vi "Controlar brazo.vi"() -> (3 "fin":bool)   [LabVIEW 2018]
panel:
  in  "Stop Button":bool
  out "Elapsed Time (s) 2":dbl
  out "Tiempo \ntranscurrido (s) 2":dbl caption="Elapsed Time (s)"
  out "Elapsed Time (s)":dbl
  out "Tiempo \ntranscurrido (s)":dbl caption="Elapsed Time (s)"
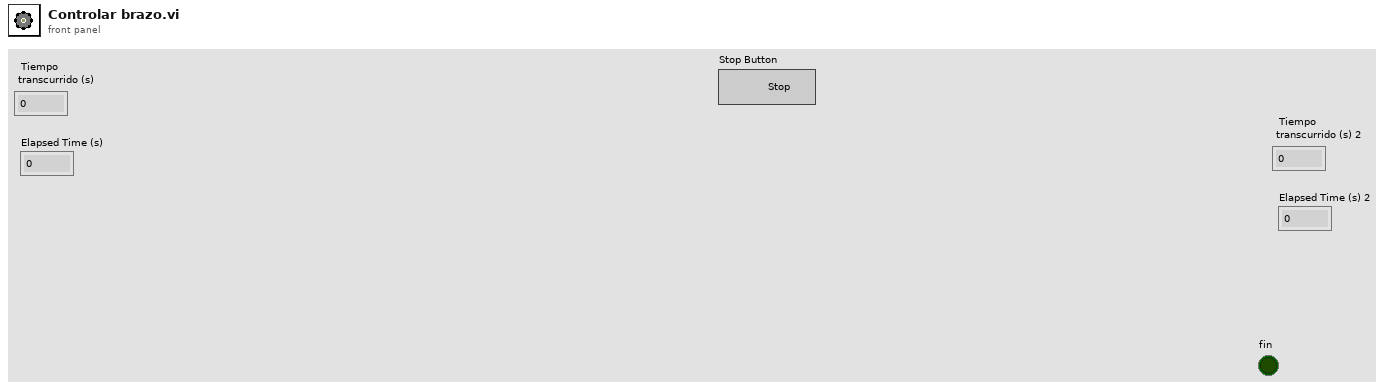
[diagram p1: front panel]
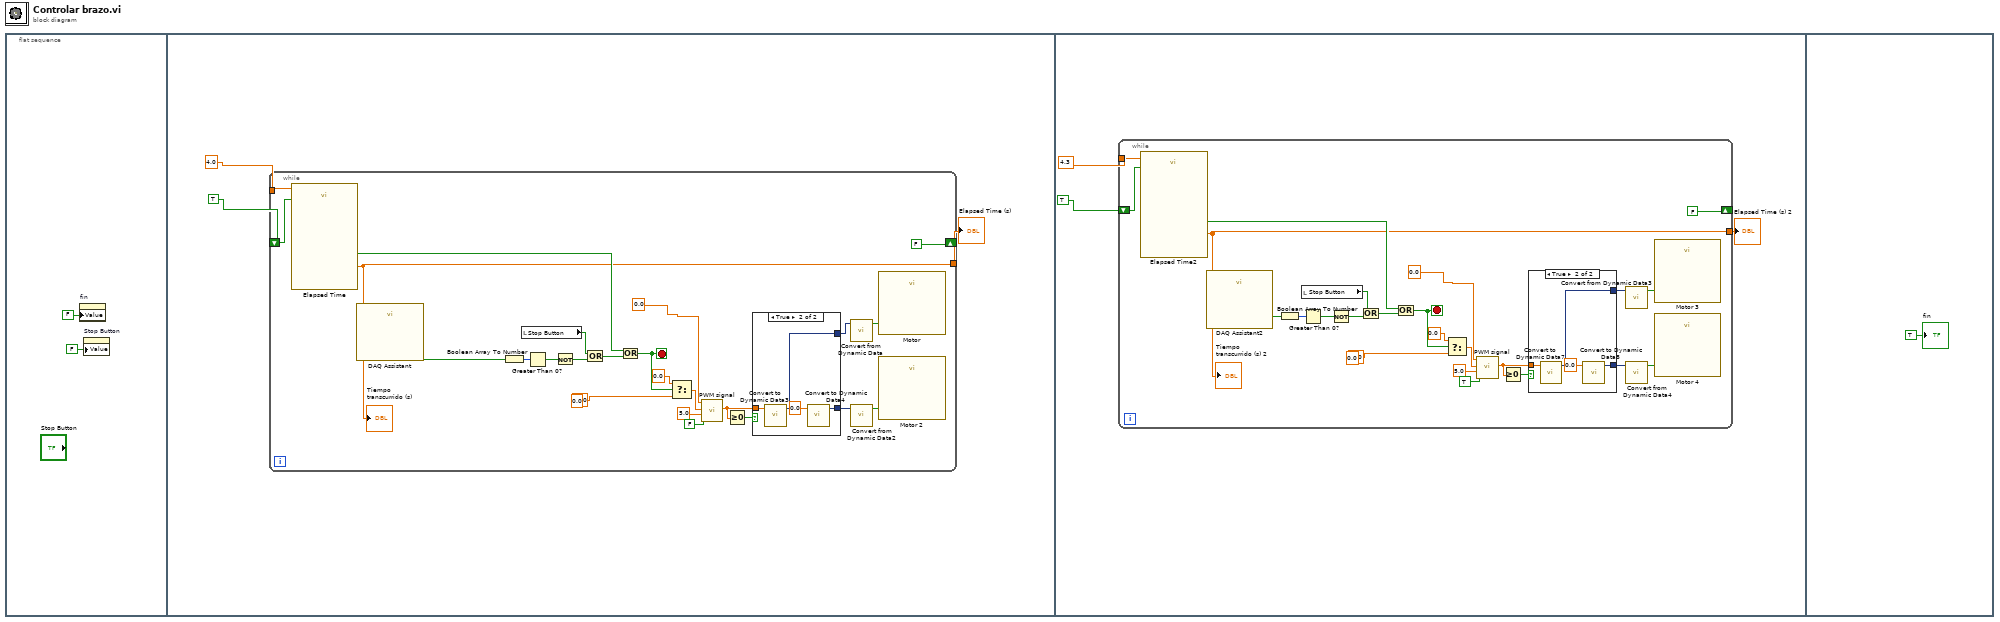
[diagram p0: block diagram]
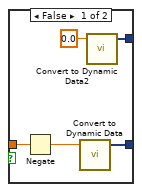
[diagram p2: hidden frame]
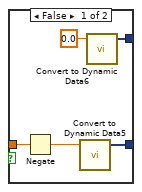
[diagram p3: hidden frame]
diagram:
  n1 = flat-sequence {
    frame #0 {
      n2 = property on="fin" class="Bool (strict)"("Value"=FALSE ("fin")) -> ()  [unwired: 2 in, 2 out]
      n3 = property on="Stop Button" class="Bool (strict)"("Value"=FALSE ("Stop Button")) -> ()  [unwired: 2 in, 2 out]
    }
    frame #1 {
      n4 = while {
        tunnel: 4.0 -> [w7]
        tunnel: [w12] -> w4
        shift-right: [FALSE] -> _
        shift-left: TRUE -> [w6]
        stop <- w16 stop-if-true
        (unwired) 0.0
        n5 = call "Elapsed Time"("Time Target (s)"=w7, "Reset"=w6) -> ("Elapsed Time (s)"=w12:dbl, "Time has Elapsed"=w17:bool)  [unwired: 10 in, 6 out]
        "Tiempo \ntranscurrido (s)" <- w12
        n6 = call "DAQ Assistant"() -> ("data"=w21:bool[])  [unwired: 17 in, 2 out]
        n7 = Boolean Array To Number(Boolean array=w21) -> (number=w20:u32)
        n8 = local read "Stop Button"() -> (w9:bool)
        n9 = Greater Than 0?(x=w20) -> (x > 0?=w19:bool)
        n10 = Not(x=w19) -> (.not. x?=w8:bool)
        n11 = Or(x=w9, y=w8) -> (x .or. y?=w18:bool)
        n12 = Or(x=w17, y=w18) -> (x .or. y?=w16:bool)
        n13 = Select(t=0.0, s=w16, f=90.0) -> (s? t:f=w22:dbl)
        n14 = call "PWM signal.vi"("Signo"=FALSE, "Amplitud"=5.0, "Ciclo de trabajo"=w22, "Frecuencia"=0.0) -> ("Waveform Chart"=w29:dbl)  [unwired: 7 in]
        n15 = Greater Or Equal To 0?(x=w29) -> (x >= 0?=w28:bool)
        n16 = case shown="True" w28 {
          tunnel: w29 -> [w31 w37]
          tunnel: [w33 w38] -> w27
          tunnel: [w34 w36] -> w25
          frame False {
            n17 = Negate(x=w31) -> (-x=w30:dbl)
            n18 = call "Convert to Dynamic Data"("Double"=w30) -> ("Dynamic Data Type"=w34:dynamicdata)  [unwired: 3 in]
            n19 = call "Convert to Dynamic Data2"("Double"=0.0) -> ("Dynamic Data Type"=w33:dynamicdata)  [unwired: 3 in]
          }
          frame True {
            n20 = call "Convert to Dynamic Data3"("Double"=w37) -> ("Dynamic Data Type"=w38:dynamicdata)  [unwired: 3 in]
            n21 = call "Convert to Dynamic Data4"("Double"=0.0) -> ("Dynamic Data Type"=w36:dynamicdata)  [unwired: 3 in]
          }
        }
        n22 = call "Convert from Dynamic Data"("Dynamic Data Type"=w27) -> ("Array"=w26:bool[])  [unwired: 3 in]
        n23 = call "Convert from Dynamic Data2"("Dynamic Data Type"=w25) -> ("Array"=w24:bool[])  [unwired: 3 in]
        n24 = call "Motor"("data"=w26) -> ()  [unwired: 17 in, 2 out]
        n25 = call "Motor 2"("data"=w24) -> ()  [unwired: 17 in, 2 out]
      }
      "Elapsed Time (s)" <- w4
    }
    frame #2 {
      n26 = while {
        tunnel: 4.3 -> [w42]
        tunnel: [w47] -> w40
        shift-right: [FALSE] -> _
        shift-left: TRUE -> [w43]
        stop <- w51 stop-if-true
        (unwired) 0.0
        n27 = call "Elapsed Time2"("Time Target (s)"=w42, "Reset"=w43) -> ("Elapsed Time (s)"=w47:dbl, "Time has Elapsed"=w52:bool)  [unwired: 10 in, 6 out]
        "Tiempo \ntranscurrido (s) 2" <- w47
        n28 = call "DAQ Assistant2"() -> ("data"=w57:bool[])  [unwired: 17 in, 2 out]
        n29 = Boolean Array To Number(Boolean array=w57) -> (number=w56:u32)
        n30 = local read "Stop Button"() -> (w44:bool)
        n31 = Greater Than 0?(x=w56) -> (x > 0?=w55:bool)
        n32 = Not(x=w55) -> (.not. x?=w54:bool)
        n33 = Or(x=w44, y=w54) -> (x .or. y?=w53:bool)
        n34 = Or(x=w52, y=w53) -> (x .or. y?=w51:bool)
        n35 = Select(t=0.0, s=w51, f=90.0) -> (s? t:f=w58:dbl)
        n36 = call "PWM signal.vi"("Signo"=TRUE, "Amplitud"=5.0, "Ciclo de trabajo"=w58, "Frecuencia"=0.0) -> ("Waveform Chart"=w65:dbl)  [unwired: 7 in]
        n37 = Greater Or Equal To 0?(x=w65) -> (x >= 0?=w64:bool)
        n38 = case shown="True" w64 {
          tunnel: w65 -> [w67 w73]
          tunnel: [w69 w74] -> w63
          tunnel: [w70 w72] -> w61
          frame False {
            n39 = Negate(x=w67) -> (-x=w66:dbl)
            n40 = call "Convert to Dynamic Data5"("Double"=w66) -> ("Dynamic Data Type"=w70:dynamicdata)  [unwired: 3 in]
            n41 = call "Convert to Dynamic Data6"("Double"=0.0) -> ("Dynamic Data Type"=w69:dynamicdata)  [unwired: 3 in]
          }
          frame True {
            n42 = call "Convert to Dynamic Data7"("Double"=w73) -> ("Dynamic Data Type"=w74:dynamicdata)  [unwired: 3 in]
            n43 = call "Convert to Dynamic Data8"("Double"=0.0) -> ("Dynamic Data Type"=w72:dynamicdata)  [unwired: 3 in]
          }
        }
        n44 = call "Convert from Dynamic Data3"("Dynamic Data Type"=w63) -> ("Array"=w62:bool[])  [unwired: 3 in]
        n45 = call "Convert from Dynamic Data4"("Dynamic Data Type"=w61) -> ("Array"=w60:bool[])  [unwired: 3 in]
        n46 = call "Motor 3"("data"=w62) -> ()  [unwired: 17 in, 2 out]
        n47 = call "Motor 4"("data"=w60) -> ()  [unwired: 17 in, 2 out]
      }
      "Elapsed Time (s) 2" <- w40
    }
    frame #3 {
      "fin" <- TRUE ("fin")
    }
  }
